vi "MDrive_Close_Com.vi"(0 "error out":errorcluster, 3 "VISA resource name in":refnum<visa-resource-name>) -> ()   [LabVIEW 2015]
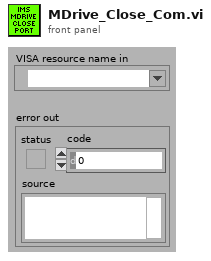
[diagram p1: front panel]
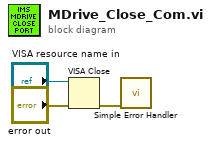
[diagram p0: block diagram]
diagram:
  n1 = VISA Close(VISA resource name="VISA resource name in", error in (no error)="error out") -> (error out=w1:errorcluster)
  n2 = call <vilib>:"Simple Error Handler.vi"("error in (no error)"=w1) -> ()  [unwired: 4 in, 5 out]
